vi "SubVi_Desactivar.vi"(10 "Indice de Alarma":i32, 11 "input cluster":T1) -> (3 "output cluster":T1)   [LabVIEW 2017]
uses:
  Cluster_Inicial.ctl
  <vilib>/Modbus/master/Modbus Master.lvclass
  <vilib>/addons/_office/excel.llb/Excel Get Data (str).vi
  <vilib>/addons/_office/excel.llb/Excel Easy Table (str).vi
  <vilib>/Utility/NIReport.llb/NI_report.lvclass
  <vilib>/addons/_office/NI_ReportGenerationToolkit.lvlib
  <vilib>/Utility/NIReport.llb/Excel/NI_Excel.lvclass
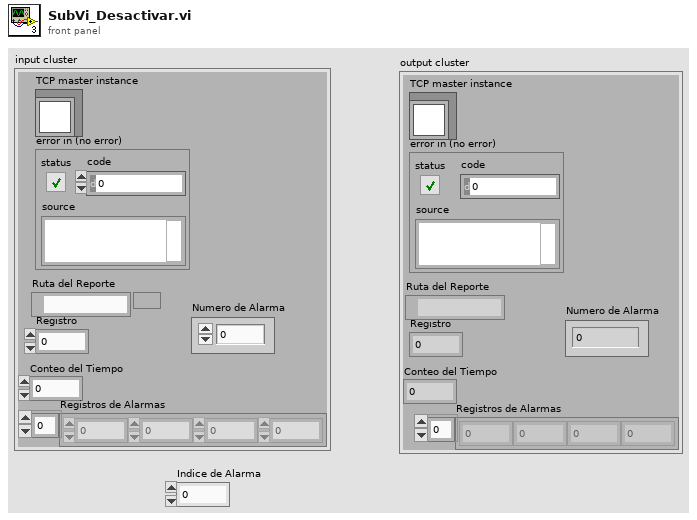
[diagram p1: front panel]
types:
  T1 = typedef "Cluster_Inicial.ctl" = cluster{"TCP master instance":refnum<class "Modbus Master.lvclass">, "error in (no error)":errorcluster, "Ruta del Reporte":path, "Registro":i32, "Conteo del Tiempo":i32, "Registros de Alarmas":i32[], "Numero de Alarma":u32}
  T2 = enum16{"maximized", "minimized", "normal", "no change"}
  T3 = enum16{"Standard Report", "HTML", "Word", "Excel"}
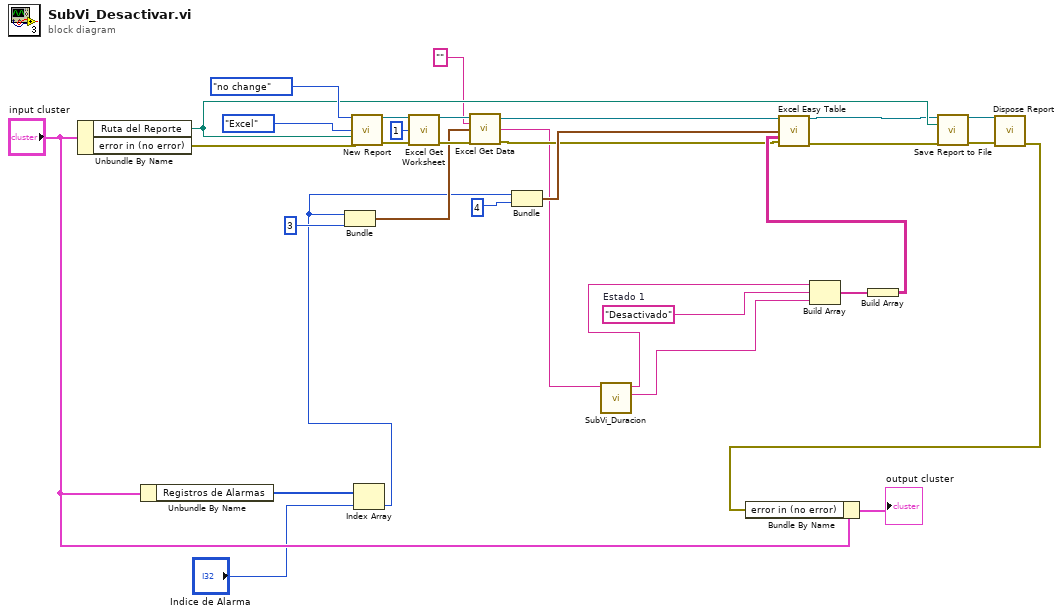
[diagram p0: block diagram]
diagram:
  w4 = "Desactivado"  # Estado 1
  n1 = Unbundle By Name("input cluster") -> ("Ruta del Reporte"=w29:path, "error in (no error)"=w26:errorcluster)
  n2 = Unbundle By Name("input cluster") -> ("Registros de Alarmas"=w15:i32[])
  n3 = call <vilib>:"New Report.vi"("window state (normal)"=T2."no change", "report type"=T3."Excel", "template (empty)"=w29, "error in (no error)"=w26) -> ("report out"=w22:refnum<class "NI_report.lvclass">, "error out"=w23:errorcluster)  [unwired: 10 in]
  n4 = Index Array(array=w15, index="Indice de Alarma") -> (element=w10:i32)
  n5 = Bundle(w10, 3) -> (w13:cluster{i32, i32})  [unwired: 1 in]
  n6 = call <vilib>:"Excel Get Worksheet.vi"("report in"=w22, "worksheet index (0)"=1, "error in (no error)"=w23) -> ("report out"=w21:refnum<class "NI_report.lvclass">, "error out"=w20:errorcluster)  [unwired: 11 in]
  n7 = call-poly <vilib>:"Excel Get Data.vi"("report in"=w21, "data type"="", "start (0, 0)"=w13, "error in (no error)"=w20) -> ("report out"=w7:refnum<class "NI_report.lvclass">, "data"=w3:string, "error out"=w8:errorcluster)  [unwired: 9 in]
  n8 = Bundle(w10, 4) -> (w9:cluster{i32, i32})  [unwired: 1 in]
  n9 = call "SubVi_Duracion.vi"("Tiempo 2"=w3) -> ("Tiempo string"=w1:string, "Duracion String"=w2:string)  [unwired: 7 in, 1 out]
  n10 = Build Array(w1, w4, w2) -> (w30:string[])
  n11 = Build Array(w30) -> (w31:string[][])
  n12 = call-poly <vilib>:"Excel Easy Table.vi"("report in"=w7, "start (0, 0)"=w9, "text data"=w31, "error in (no error)"=w8) -> ("report out"=w5:refnum<class "NI_report.lvclass">, "error out"=w6:errorcluster)  [unwired: 7 in, 3 out]
  n13 = call-dynamic "Save Report to File.vi"("report in"=w5, "report file path"=w29, "error in (no error)"=w6) -> ("report out"=w27:refnum<class "NI_report.lvclass">, "error out"=w28:errorcluster)  [unwired: 11 in]
  n14 = call-dynamic "Dispose Report.vi"("report in"=w27, "error in (no error)"=w28) -> ("error out"=w17:errorcluster)  [unwired: 13 in]
  n15 = Bundle By Name(cluster="input cluster", "error in (no error)"=w17) -> (→"output cluster":T1)
